vi "traceSnapTest.vi"() -> ()   [LabVIEW 2012]
uses:
  <vilib>/userdefined/High Color/IMAQdx.ctl
  <vilib>/vision/Image Controls.llb/IMAQ Image.ctl
  <vilib>/vision/driver/NI_Vision_Acquisition_Software.lvlib
  <vilib>/vision/NI_Vision_Development_Module.lvlib
panel:
  out "Image Out":T1(plugin-control)
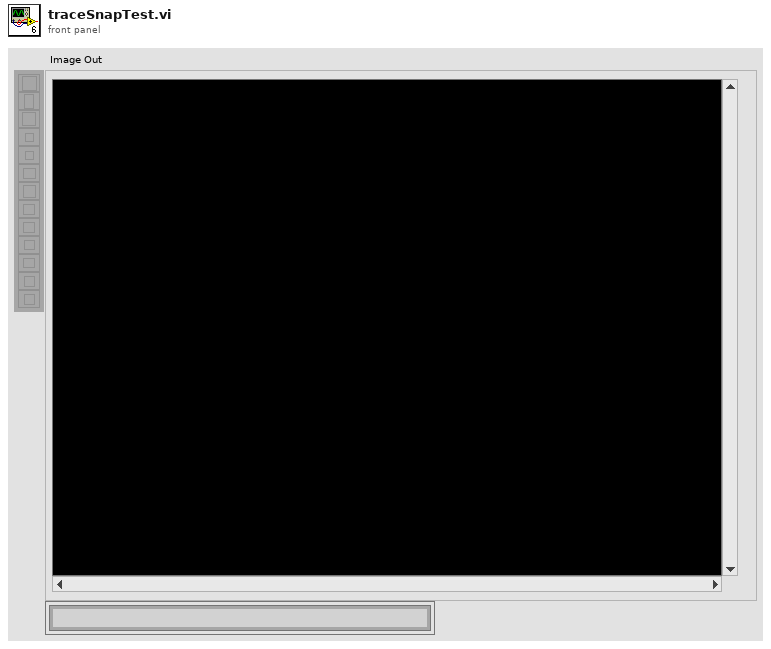
[diagram p1: front panel]
types:
  T1 = typedef "IMAQ Image.ctl" = refnum<image>
  T2 = typedef "Image Type" = u32
  T3 = cluster{"Number of Matches Requested":i32, "Minimum Match Score":sgl, "Angle Ranges":cluster{"Start Angle":sgl, "End Angle":sgl}[]}
  T4 = typedef "IMAQdx.ctl" = refnum<k21>
  T5 = typedef "IMAQ Rectangle" = cluster{"Left":i32, "Top":i32, "Right":i32, "Bottom":i32, "Rotation":dbl}
  T6 = typedef "ROI Descriptor" = cluster{"Global Rectangle":i32[], "Contours":cluster{"ID":enum32{"External", "Internal"}, "Type":u32, "Coordinates":i32[]}[]}
  T7 = cluster{"Position":cluster{"x":sgl, "y":sgl}, "Angle":sgl, "Scale":sgl, "Score":sgl, "Bounding Box":cluster{"x":sgl, "y":sgl}[]}[]
  T8 = cluster{"Matches (real-world)[0]":cluster{"Position":cluster{"x":sgl, "y":sgl}, "Angle":sgl, "Scale":sgl, "Score":sgl, "Bounding Box":cluster{"x":sgl, "y":sgl}[]}, "Matches (real-world)[1]":cluster{"Position":cluster{"x":sgl, "y":sgl}, "Angle":sgl, "Scale":sgl, "Score":sgl, "Bounding Box":cluster{"x":sgl, "y":sgl}[]}, "Matches (real-world)[2]":cluster{"Position":cluster{"x":sgl, "y":sgl}, "Angle":sgl, "Scale":sgl, "Score":sgl, "Bounding Box":cluster{"x":sgl, "y":sgl}[]}, "Matches (real-world)[3]":cluster{"Position":cluster{"x":sgl, "y":sgl}, "Angle":sgl, "Scale":sgl, "Score":sgl, "Bounding Box":cluster{"x":sgl, "y":sgl}[]}}
  T9 = cluster{"Bounding Box[0]":cluster{"x":sgl, "y":sgl}, "Bounding Box[1]":cluster{"x":sgl, "y":sgl}, "Bounding Box[2]":cluster{"x":sgl, "y":sgl}, "Bounding Box[3]":cluster{"x":sgl, "y":sgl}, "Bounding Box[4]":cluster{"x":sgl, "y":sgl}, "Bounding Box[5]":cluster{"x":sgl, "y":sgl}, "Bounding Box[6]":cluster{"x":sgl, "y":sgl}, "Bounding Box[7]":cluster{"x":sgl, "y":sgl}, "Bounding Box[8]":cluster{"x":sgl, "y":sgl}}
  T10 = cluster{"[0]":sgl, "[1]":sgl, "[2]":sgl, "[3]":sgl}
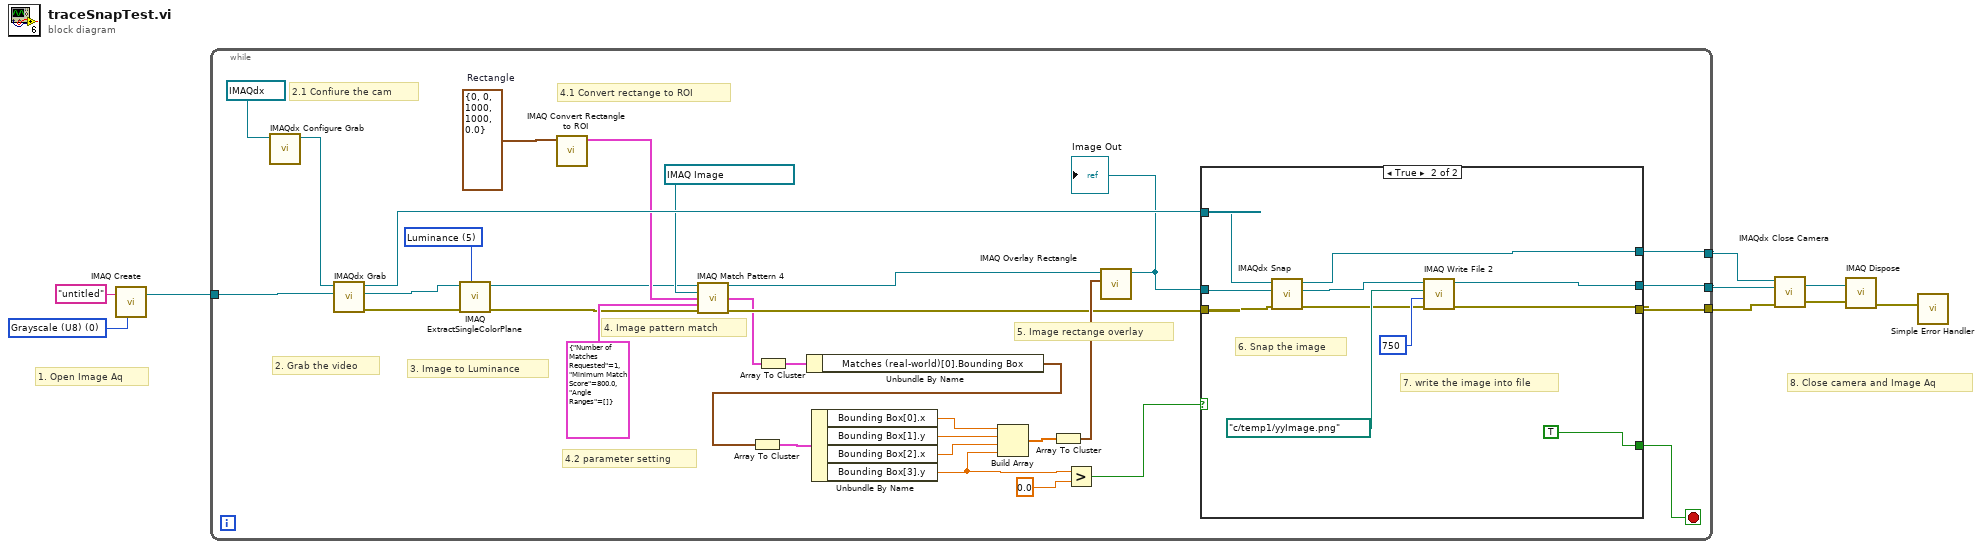
[diagram p0: block diagram]
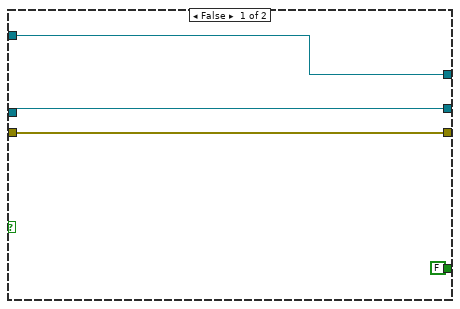
[diagram p2: hidden frame]
diagram:
  w7 = T2 0 items=["Grayscale (U8)", "Grayscale (I16)", "Grayscale (SGL)", "Complex (CSG)", "RGB (U32)", "HSL (U32)", "RGB (U64)", "Grayscale (U16)"] ("Image Type")
  # "8. Close camera and Image Aq"
  # "1. Open Image Aq"
  n1 = call "IMAQ Create"("Image Name"="untitled", "Image Type"=w7) -> ("New Image"=w6:T1)  [unwired: 3 in, 1 out]
  n2 = while {
    tunnel: w6 -> [w39]
    tunnel: [w25] -> w3
    tunnel: [w24] -> w2
    tunnel: [w22] -> w1
    stop <- w21 stop-if-true
    w9 = 5 items=["Red", "Green", "Blue", "Hue", "Saturation", "Luminance", "Value", "Intensity"] ("Color Plane")
    w16 = T5 {"Left"=0, "Top"=0, "Right"=1000, "Bottom"=1000, "Rotation"=0.0}  # Rectangle
    # "4.2 parameter setting"
    # "4.1 Convert rectange to ROI"
    # "2.1 Confiure the cam"
    # "5. Image rectange overlay"
    # "4. Image pattern match"
    # "3. Image to Luminance"
    # "2. Grab the video"
    n3 = call <vilib>:"IMAQdx Configure Grab.vi"("Session In"=T4 "cam0") -> ("Session Out"=w40:T4)  [unwired: 9 in, 1 out]
    n4 = call <vilib>:"IMAQdx Grab.vi"("Image In"=w39, "Session In"=w40) -> ("error out"=w11:errorcluster, "Image Out"=w13:T1, "Session Out"=w26:T4)  [unwired: 6 in, 1 out]
    n5 = call "IMAQ ExtractSingleColorPlane"("Color Plane"=w9, "error in (no error)"=w11, "Image Src"=w13) -> ("error out"=w10:errorcluster, "Image Dst Out"=w12:T1)  [unwired: 7 in]
    n6 = call "IMAQ Convert Rectangle to ROI"("Rectangle"=w16) -> ("ROI Descriptor"=w15:T6)  [unwired: 8 in, 1 out]
    n7 = call "IMAQ Match Pattern 4"("Image"=w12, "Template Image"=T1 refnum, "ROI Descriptor"=w15, "Parameters"=T3 {"Number of Matches Requested"=1, "Minimum Match Score"=800.0, "Angle Ranges"=[]}, "error in (no error)"=w10) -> ("Image (duplicate)"=w18:T1, "Matches (real-world)"=w17:T7, "error out"=w20:errorcluster)  [unwired: 6 in, 2 out]
    n8 = Array To Cluster(array=w17) -> (cluster=w38:T8)
    n9 = Unbundle By Name(w38) -> ("Matches (real-world)[0].Bounding Box"=w37:cluster{"x":sgl, "y":sgl}[])
    n10 = Array To Cluster(array=w37) -> (cluster=w36:T9)
    n11 = Unbundle By Name(w36) -> ("Bounding Box[0].x"=w35:sgl, "Bounding Box[1].y"=w34:sgl, "Bounding Box[2].x"=w33:sgl, "Bounding Box[3].y"=w29:sgl)
    n12 = Build Array(w35, w34, w33, w29) -> (w32:sgl[])
    n13 = Array To Cluster(array=w32) -> (cluster=w31:T10)
    n14 = Greater?(x=w29, y=sgl 0.0) -> (0:w27:bool)
    n15 = call "IMAQ Overlay Rectangle"("Rectangle"=w31, "Image"=w18) -> ("Image Out"=w23:T1)  [unwired: 8 in, 1 out]
    "Image Out" <- w23
    n16 = case shown="True" w27 {
      tunnel: w26 -> [w44 w55]
      tunnel: [w44 w54] -> w25
      tunnel: w20 -> [w43 w53]
      tunnel: [w43 w46] -> w24
      tunnel: w23 -> [w42 w52]
      tunnel: [w42 w48] -> w22
      tunnel: [FALSE TRUE] -> w21
      frame False {
      }
      frame True {
        # "7. write the image into file"
        # "6. Snap the image"
        n17 = call <vilib>:"IMAQdx Snap.vi"("error in"=w53, "Image In"=w52, "Session In"=w55) -> ("error out"=w47:errorcluster, "Image Out"=w50:T1, "Session Out"=w54:T4)  [unwired: 6 in]
        n18 = call-poly "IMAQ Write File 2"("error in (no error)"=w47, "Image Quality"=u32 750, "File Path"=path "c:/temp1/yyImage.png", "Image"=w50) -> ("error out"=w46:errorcluster, "Image Out (duplicate)"=w48:T1)  [unwired: 6 in]
      }
    }
  }
  n19 = call <vilib>:"IMAQdx Close Camera.vi"("error in"=w2, "Session In"=w3) -> ("error out"=w5:errorcluster)  [unwired: 9 in]
  n20 = call "IMAQ Dispose"("Image"=w1, "error in (no error)"=w5) -> ("error out"=w4:errorcluster)  [unwired: 1 in, 3 out]
  n21 = call <vilib>:"Simple Error Handler.vi"("error in (no error)"=w4) -> ()  [unwired: 1 in, 8 out]
